vi "Delete.vi"(6 "Index in":i32, 8 "error in (no error)":errorcluster, 11 "Composite Object in":refnum<class "CConfig Object.lvclass">) -> (0 "error out":errorcluster, 2 "Deleted?":bool, 3 "Composite Object out":refnum<class "CConfig Object.lvclass">, 4 "Index in":i32)   [LabVIEW 2013, in "CConfig Object.lvclass"]
doc: "Copyright 2018, Carya Automatisering, Wiebe Walstra."
uses:
  CConfig Object.lvclass
  CConfig Object.lvclass/CConfig Object.ctl
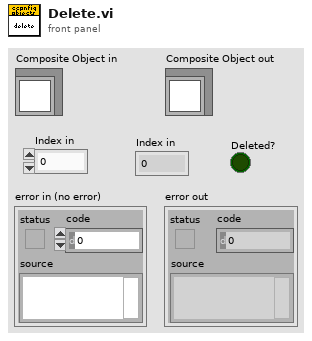
[diagram p1: front panel]
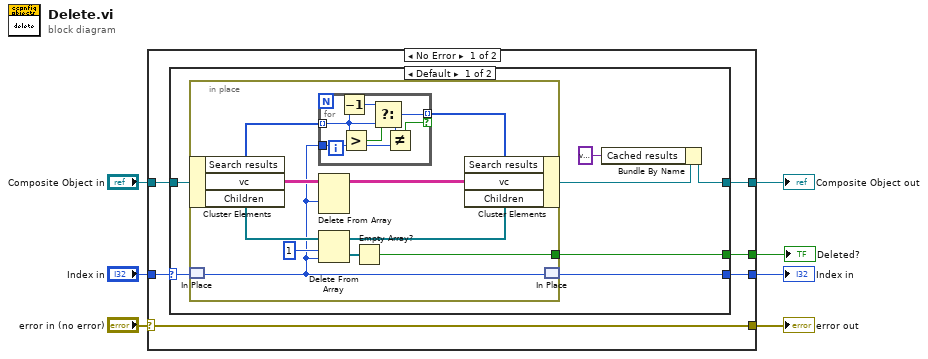
[diagram p0: block diagram]
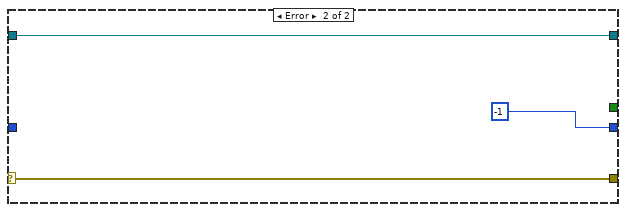
[diagram p3: hidden frame]
diagram:
  n1 = case shown="No Error" "error in (no error)" {
    selector: "error in (no error)" -> [w13 w41]
    tunnel: [w13 w41] -> w6
    tunnel: [w11 w40] -> w4
    tunnel: "Composite Object in" -> [w12 w40]
    tunnel: "Index in" -> [w10 _]
    tunnel: [w9 -1 ("Index in")] -> w2
    tunnel: [w8 _] -> w1
    frame No Error {
      n2 = case shown="Default" w10 {
        selector: w10 -> [w15 w38]
        tunnel: w12 -> [w20 w37]
        tunnel: [w16 w37] -> w11
        tunnel: [w14 w38] -> w9
        tunnel: [w19 _] -> w8
        frame Default {
          n3 = in-place {
            in-place-border: [w24] -> w19
            n4 = in-place-cluster #1(w20) -> ("Search results"=w23:i32[], "vc"=w30:string[][], "Children"=w28:refnum<class>[])
            n5 = in-place-match #2(w15) -> (w21:i32)
            n6 = for {
              tunnel: [w35] -> w22 mode=indexing if=w31
              tunnel: w23 -> [w32] mode=indexing
              tunnel: w21 -> [w33]
              n7 = Decrement(x=w32) -> (x-1=w36:i32)
              n8 = Greater?(x=w32, y=w33) -> (0:w34:bool)
              n9 = Select(t=w36, s=w34, f=w32) -> (s? t:f=w35:i32)
              n10 = Not Equal?(x=w32, y=w33) -> (x != y?=w31:bool)
            }
            n11 = Delete From Array(array=w30, index (row)=w21) -> (array with subset deleted=w29:string[][])  [unwired: 2 in, 1 out]
            n12 = Delete From Array(array=w28, length=1, index=w21) -> (deleted portion=w25:refnum<class>[], array with subset deleted=w27:refnum<class>[])
            n13 = Empty Array?(array=w25) -> (empty?=w24:bool)
            n14 = in-place-cluster #1("Search results"=w22, "vc"=w29, "Children"=w27) -> (w17:refnum<class "CConfig Object.lvclass">)
            n15 = in-place-match #2(w21) -> (w14:i32)
          }
          n16 = Bundle By Name(cluster=w17, "Cached results"=variant) -> (w16:refnum<class "CConfig Object.lvclass">)
        }
        frame -1 {
        }
      }
    }
    frame Error {
    }
  }
  "error out" <- w6
  "Composite Object out" <- w4
  "Index in" <- w2
  "Deleted?" <- w1
